vi "Default Configuration.vi"() -> (3 "DAQmx Configuration":T1 {"Run Mode" items=["Run Once", "Continuously"]; "Block Size" min=0; "Sample Rate (Hz)" min=0.0; "Trigger Type" items=["None", "Analog Reference"]; "Channel Table"."input terminal configuration" items=["default"=-1, "RSE"=10083, "NRSE"=10078, "Differential"=10106, "Pseudodifferential"=12529]; "Channel Table"."Channel Type" items=["Voltage (V)"=0, "Charge (C)"=9, "-"=99, "SPL (Pa)"=3, "Force (lbf)"=6, "Force (N)"=1, "Acceleration (g) - IEPE"=2, "Acceleration (g) - Charge"=12, "Acceleration (g) - 4 wire DC Voltage"=22, "Velocity (in/s)"=7, "Velocity (mm/s)"=8, "Prox Probe (mil)"=4, "Prox Probe (mm)"=5]})   [LabVIEW 2024, in "Dynamic Signal Acquisition (Interactive) UI.lvlib"]
uses:
  Dynamic Signal Acquisition (Interactive) UI.lvlib
  SFPDAQ Configuration.ctl
  SFPDAQmx Channel Info.ctl
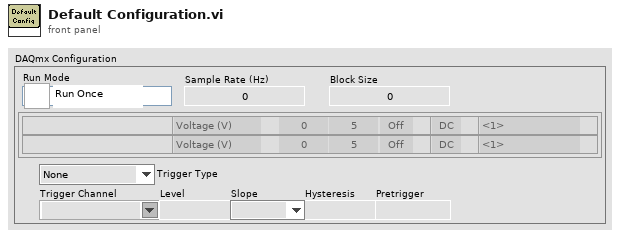
[diagram p1: front panel]
types:
  T1 = typedef "Dynamic Signal Acquisition (Interactive) UI.lvlib/SFPDAQ Configuration.ctl" = cluster{"Run Mode":u16, "Sample Rate (Hz)":dbl, "Block Size":i32, "Channel Table":T2[], "Trigger Type":u16, "Trigger Channel":string, "Level":dbl, "Pretrigger":i32, "Hysteresis":dbl, "Slope":enum16{"Falling", "Rising"}}
  T2 = typedef "Dynamic Signal Acquisition (Interactive) UI.lvlib/SFPDAQmx Channel Info.ctl" = cluster{"DAQmx Channel":tag, "Channel Type":u16, "Max":dbl, "Sensitivity":dbl, "Coupling":enum16{"AC", "DC"}, "input terminal configuration":i32, "excitation":enum16{"Off", "Min", "Max"}}
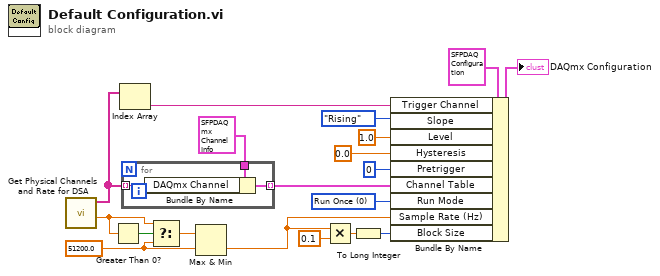
[diagram p0: block diagram]
diagram:
  w18 = u16 0 items=["Run Once", "Continuously"] ("Run Mode")
  w3 = 51200.0 ("Sample Rate (Hz)")
  n1 = call "Get Physical Channels and Rate for DSA.vi"() -> ("maximum rate"=w6:dbl, "physical channels"=w13:tag[])  [unwired: 10 in]
  n2 = Greater Than 0?(x=w6) -> (x > 0?=w1:bool)
  n3 = Index Array(array=w13) -> (element=w8:tag)  [unwired: 1 in]
  n4 = for {
    tunnel: w13 -> [w22] mode=indexing
    tunnel: T2 {"DAQmx Channel"="", "Channel Type"=0, "Max"=5.0, "Sensitivity"=1000.0, "Coupling"=enum."DC", "input terminal configuration"=-1, "excitation"=enum."Off"} ("Channel Information") -> [w21]
    tunnel: [w20] -> w15 mode=indexing
    n5 = Bundle By Name(cluster=w21, "DAQmx Channel"=w22) -> (w20:T2)
  }
  n6 = Select(t=w6, s=w1, f=w3) -> (s? t:f=w2:dbl)
  n7 = Max & Min(x=w2, y=w3) -> (min(x,y)=w16:dbl)  [unwired: 1 out]
  n8 = Multiply(x=w16, y=0.1 ("Sample Rate (Hz)")) -> (x*y=w5:dbl)
  n9 = To Long Integer(number=w5) -> (32bit integer=w17:i32)
  n10 = Bundle By Name(cluster=T1 {"Run Mode"=0, "Sample Rate (Hz)"=51200.0, "Block Size"=5120, "Channel Table"=[], "Trigger Type"=0, "Trigger Channel"="", "Level"=1.0, "Pretrigger"=20, "Hysteresis"=0.0, "Slope"=enum."Rising"} ("DAQmx Configuration"), "Trigger Channel"=w8, "Slope"=enum16{"Falling", "Rising"}."Rising", "Level"=1.0, "Hysteresis"=0.0, "Pretrigger"=0, "Channel Table"=w15, "Run Mode"=w18, "Sample Rate (Hz)"=w16, "Block Size"=w17) -> (→"DAQmx Configuration":T1)
